vi "niRFUtil MASMT 1D Convolution (CDB).vi"(6 "output size":i32(ring) items=["Full", "Size X", "Compact"], 8 "error in (no error)":errorcluster, 9 "algorithm":i32(ring)=1 items=["Direct", "Frequency Domain"], 10 "Y":cdb[](array[numeric]), 11 "X":cdb[](array[numeric])) -> (0 "error out":errorcluster, 3 "X * Y":cdb[](array[numeric]))   [LabVIEW 2016, in "niRFUtil.lvlib"]
doc: "Computes the convolution of the input sequences <B>X</B> and <B>Y</B>."
uses:
  niRFUtil.lvlib
  Utilities/niRFMASMT_FFT.dll
panel:
  out "FreqWorkH":cdb[](array[numeric])
  out "WorkH":cdb[](array[numeric])
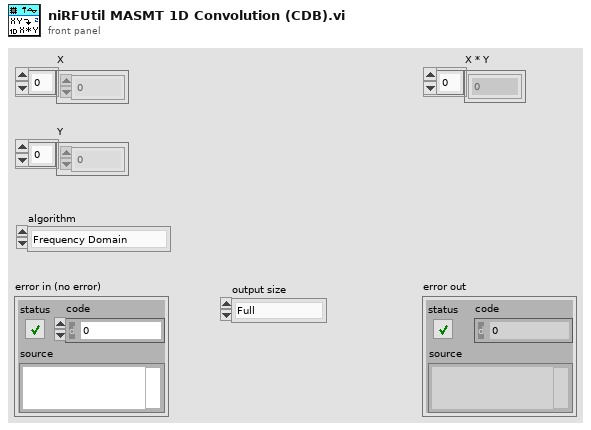
[diagram p1: front panel]
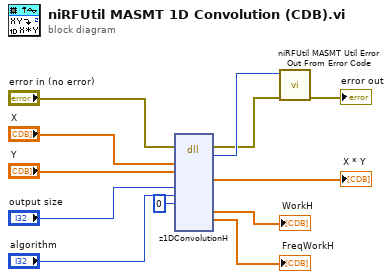
[diagram p0: block diagram]
diagram:
  n1 = dll-call lib="C:/Perforce/semoore-sales/Customers/NATI-3813/Multisite/tools/filters/niRFUtil/MASMT/Utilities/niRFMASMT_FFT.*" fn="z1DConvolutionH"(error in="error in (no error)", "X"="X", "Y"="Y", "size"="output size", "domain"="algorithm", "step"=0) -> (error out=w5:errorcluster, "error"=w7:i32, "X * Y"=→"X * Y":cdb[], "WorkH"=→"WorkH":cdb[], "FreqWorkH"=→"FreqWorkH":cdb[])  [unwired: 12 in, 1 out]
  n2 = call "niRFUtil MASMT Util Error Out From Error Code.vi"("error in (no error)"=w5, "error code"=w7) -> ("error out"=→"error out":errorcluster)  [unwired: 9 in]
